vi "PSTRA-Params To Info String.vi"(7 "PSTR Params":T1={"Stimulus"={"Ear"=enum."Right", "BW (oct)"=0.0, "Seed"=0, "Ramp (ms)"=0.0, "On time (ms)"=0.0, "Off time (ms)"=0.0, "Delay (ms)"=10000.0}, "FreqSeq"={"Min (kHz)"=0.0, "Max (kHz)"=0.0, "Step (oct)"=0.0}, "LevelSeq"={"Min (dB)"=0.0, "Max (dB)"=0.0, "Step (dB)"=0.0}, "Seq"={"Order"=enum."Sequential", "Averages"=0}, "Response"={"Grass gain"=0.0, "Window (ms)"=0.0}, "Hidden"={"Sample rate (Hz)"=0.0, "Nfft"=0, "save raw"=FALSE, "sep"=0.0, "Window"=enum."NONE"}, "RejThr"=0.0}) -> (8 "Info":string)   [LabVIEW 2020]
uses:
  PSTR VIs/Typedefs/PSTR-Parameters.ctl
  PSTR VIs/Typedefs/PSTR-Stimulus Params.ctl
  Utility VIs/Type Defs/Left-Right ring.ctl
  PSTR VIs/Typedefs/PSTR-FreqSeq Params.ctl
  PSTR VIs/Typedefs/PSTR-LevelSeq Params.ctl
  PSTR VIs/Typedefs/PSTR-SeqParams.ctl
  PSTR VIs/Typedefs/PSTR-Response Params.ctl
  PSTR VIs/Typedefs/PSTR-Hidden Params.ctl
  PSTR VIs/Typedefs/PSTR-Window Shape.ctl
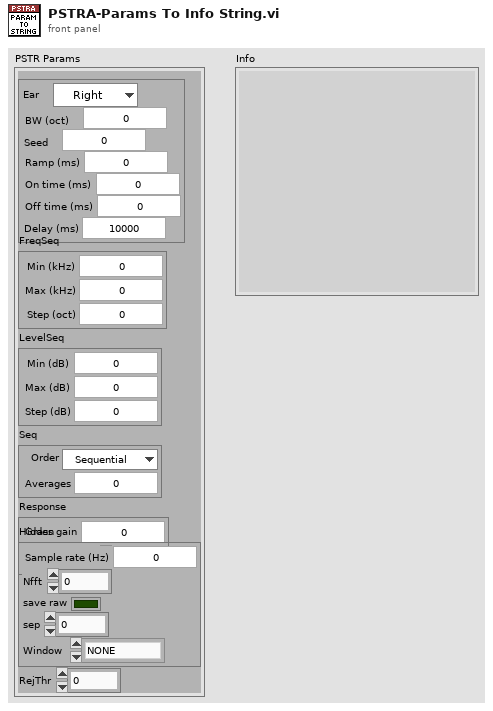
[diagram p1: front panel]
types:
  T1 = typedef "PSTR-Parameters.ctl" = cluster{"Stimulus":T2, "FreqSeq":T4, "LevelSeq":T5, "Seq":T6, "Response":T7, "Hidden":T8, "RejThr":dbl}
  T2 = typedef "PSTR-Stimulus Params.ctl" = cluster{"Ear":T3, "BW (oct)":dbl, "Seed":i32, "Ramp (ms)":dbl, "On time (ms)":dbl, "Off time (ms)":dbl, "Delay (ms)":dbl}
  T3 = typedef "Left-Right ring.ctl" = enum16{"Right", "Left"}
  T4 = typedef "PSTR-FreqSeq Params.ctl" = cluster{"Min (kHz)":dbl, "Max (kHz)":dbl, "Step (oct)":dbl}
  T5 = typedef "PSTR-LevelSeq Params.ctl" = cluster{"Min (dB)":dbl, "Max (dB)":dbl, "Step (dB)":dbl}
  T6 = typedef "PSTR-SeqParams.ctl" = cluster{"Order":enum16{"Sequential", "Random"}, "Averages":i32}
  T7 = typedef "PSTR-Response Params.ctl" = cluster{"Grass gain":dbl, "Window (ms)":dbl}
  T8 = typedef "PSTR-Hidden Params.ctl" = cluster{"Sample rate (Hz)":dbl, "Nfft":i32, "save raw":bool, "sep":dbl, "Window":T9}
  T9 = typedef "PSTR-Window Shape.ctl" = enum16{"NONE", "Hamming"}
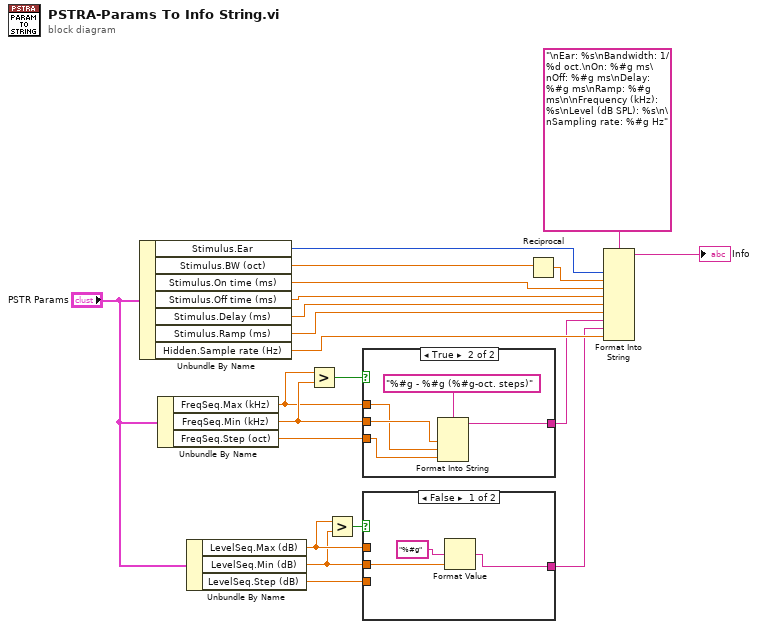
[diagram p0: block diagram]
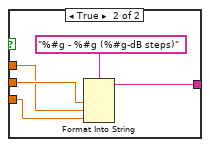
[diagram p2: hidden frame]
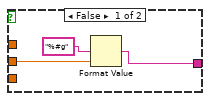
[diagram p3: hidden frame]
diagram:
  n1 = Unbundle By Name("PSTR Params") -> ("Stimulus.Ear"=w20:T3, "Stimulus.BW (oct)"=w18:dbl, "Stimulus.On time (ms)"=w17:dbl, "Stimulus.Off time (ms)"=w16:dbl, "Stimulus.Delay (ms)"=w5:dbl, "Stimulus.Ramp (ms)"=w4:dbl, "Hidden.Sample rate (Hz)"=w3:dbl)
  n2 = Unbundle By Name("PSTR Params") -> ("FreqSeq.Max (kHz)"=w12:dbl, "FreqSeq.Min (kHz)"=w13:dbl, "FreqSeq.Step (oct)"=w11:dbl)
  n3 = Unbundle By Name("PSTR Params") -> ("LevelSeq.Max (dB)"=w8:dbl, "LevelSeq.Min (dB)"=w7:dbl, "LevelSeq.Step (dB)"=w9:dbl)
  n4 = Greater?(x=w12, y=w13) -> (0:w14:bool)
  n5 = Greater?(x=w8, y=w7) -> (0:w6:bool)
  n6 = case shown="True" w14 {
    tunnel: w13 -> [w24 w28]
    tunnel: w12 -> [_ w27]
    tunnel: w11 -> [_ w26]
    tunnel: [w23 w25] -> w1
    frame False {
      n7 = Format Value(format string="%#g", value (0)=w24) -> (output string=w23:string)  [unwired: 1 in]
    }
    frame True {
      n8 = Format Into String(format string="%#g - %#g (%#g-oct. steps)", w28, w27, w26) -> (resulting string=w25:string)  [unwired: 2 in, 1 out]
    }
  }
  n9 = case shown="False" w6 {
    tunnel: w7 -> [w32 w36]
    tunnel: w8 -> [_ w35]
    tunnel: w9 -> [_ w34]
    tunnel: [w31 w33] -> w2
    frame False {
      n10 = Format Value(format string="%#g", value (0)=w32) -> (output string=w31:string)  [unwired: 1 in]
    }
    frame True {
      n11 = Format Into String(format string="%#g - %#g (%#g-dB steps)", w36, w35, w34) -> (resulting string=w33:string)  [unwired: 2 in, 1 out]
    }
  }
  n12 = Reciprocal(x=w18) -> (1/x=w19:dbl)
  n13 = Format Into String(format string="\nEar: %s\nBandwidth: 1/%d oct.\nOn: %#g ms\nOff: %#g ms\nDelay: %#g ms\nRamp: %#g ms\n\nFrequency (kHz): %s\nLevel (dB SPL): %s\n\nSampling rate: %#g Hz", w20, w19, w17, w16, w5, w4, w1, w2, w3) -> (resulting string=→"Info":string)  [unwired: 2 in, 1 out]
